vi "HeatFlow HW Conf Load.vi"(11 "Conf File":path) -> (0 "error out":errorcluster, 3 "HeatFlow HW Cfg":T1)   [LabVIEW 2019, in "Acquisition.lvlib"]
uses:
  Acquisition.lvlib
  HeatFlow HW Cfg.ctl
  HeatFlow Acq States.ctl
  <vilib>/Utility/config.llb/Read Key (Boolean).vi
  <vilib>/Utility/config.llb/Read Key (Double).vi
  <vilib>/Utility/config.llb/Read Key (String).vi
  <vilib>/Utility/config.llb/NI_LVConfig.lvlib
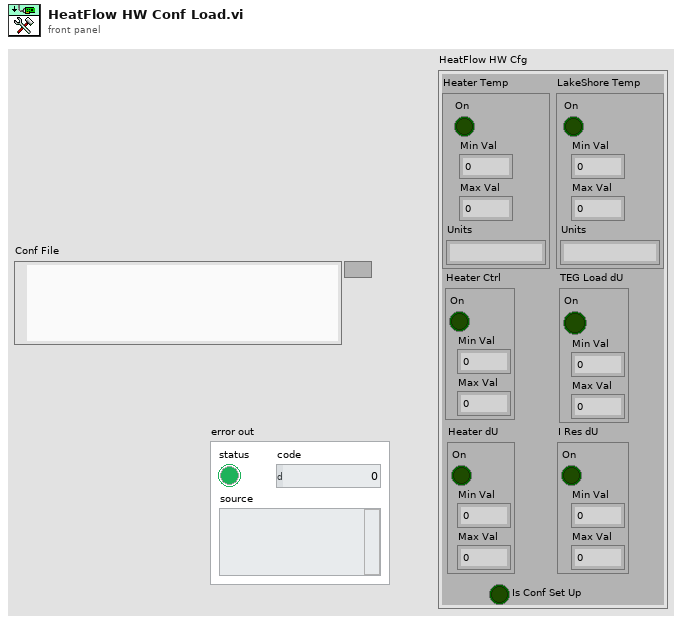
[diagram p1: front panel]
types:
  T1 = typedef "Acquisition.lvlib/HeatFlow HW Cfg.ctl" = cluster{"Heater Temp":cluster{"On":bool, "Min Val":dbl, "Max Val":dbl, "Units":string}, "LakeShore Temp":cluster{"On":bool, "Min Val":dbl, "Max Val":dbl, "Units":string}, "Heater Ctrl":cluster{"On":bool, "Min Val":dbl, "Max Val":dbl}, "TEG Load dU":cluster{"On":bool, "Min Val":dbl, "Max Val":dbl}, "Heater dU":cluster{"On":bool, "Min Val":dbl, "Max Val":dbl}, "I Res dU":cluster{"On":bool, "Min Val":dbl, "Max Val":dbl}, "Is Conf Set Up":bool}
  T2 = typedef "Acquisition.lvlib/HeatFlow Acq States.ctl" = enum16{"Start", "--- Control ---", "HeaterTemp", "DoControl?", "HeaterCtrl", "--- Readings ---", "DoReadings?", "I_Res_dU", "LakeShoreTemp", "Heater_dU", "TEG_Load_dU", "Calculations", "End"}
  T3 = typedef "NI_LVConfig.lvlib/Config Data RefNum.ctl" = refnum<k1>
  T4 = cluster{"On":bool, "Min Val":dbl, "Max Val":dbl, "Units":string}
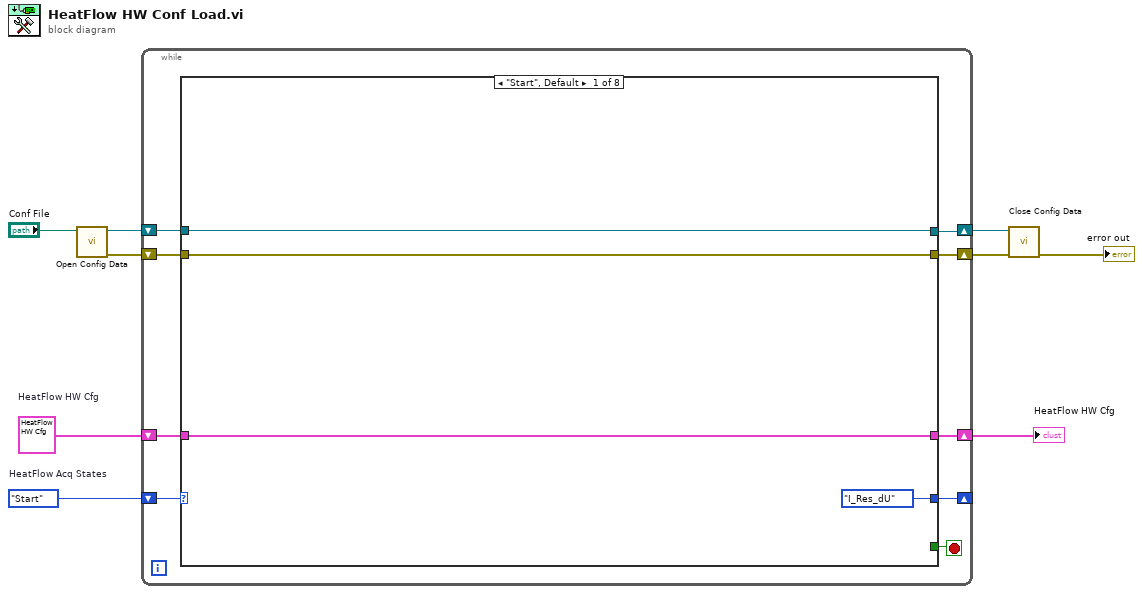
[diagram p0: block diagram]
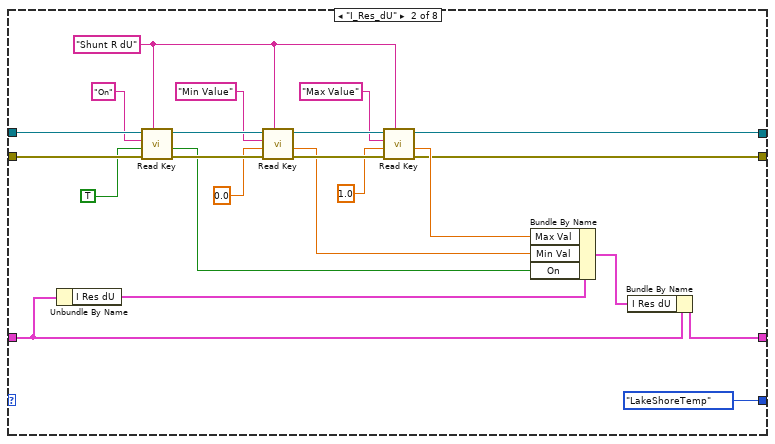
[diagram p2: hidden frame]
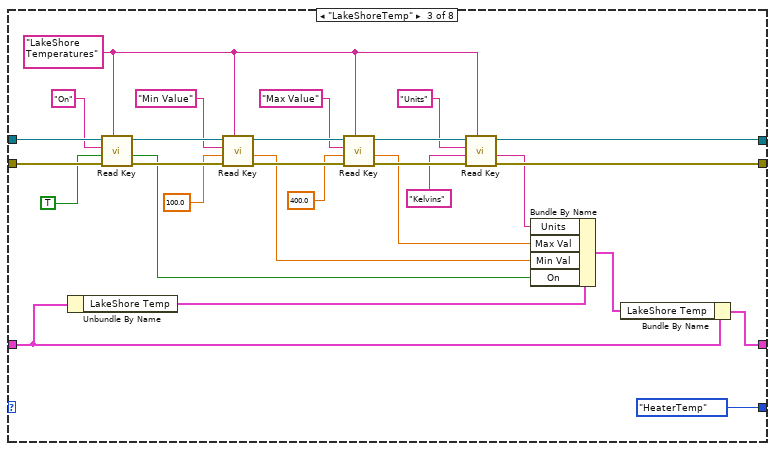
[diagram p3: hidden frame]
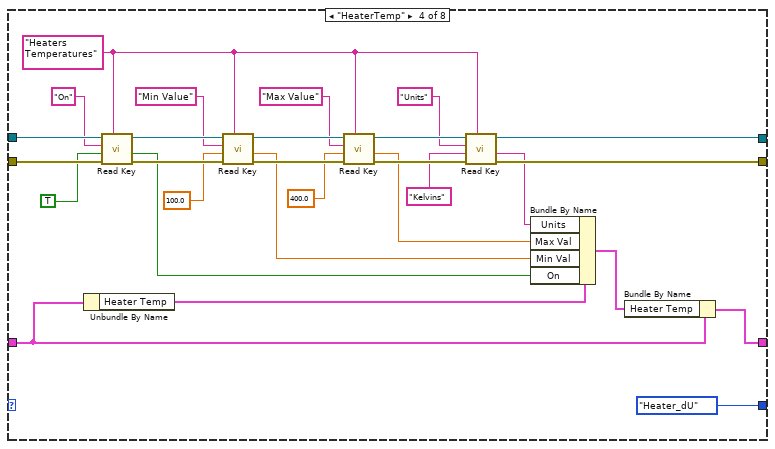
[diagram p4: hidden frame]
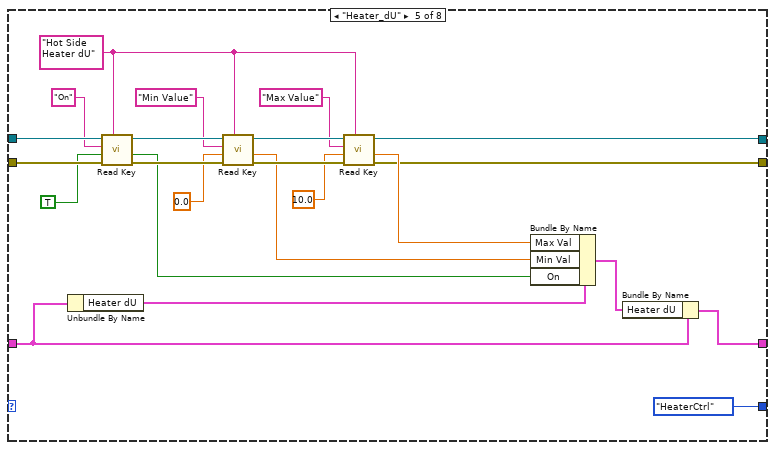
[diagram p5: hidden frame]
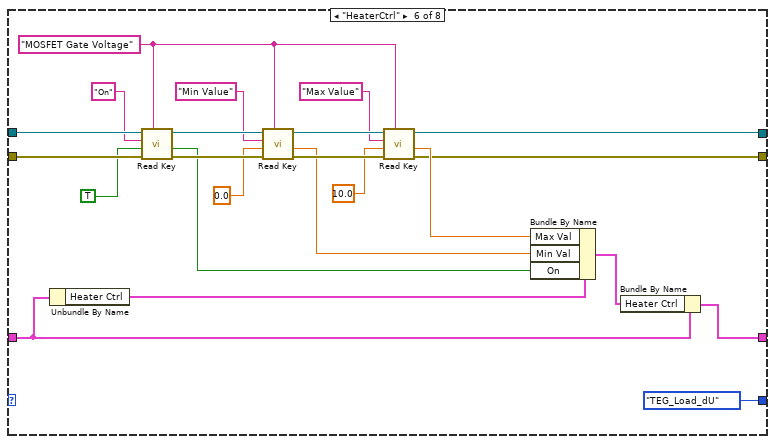
[diagram p6: hidden frame]
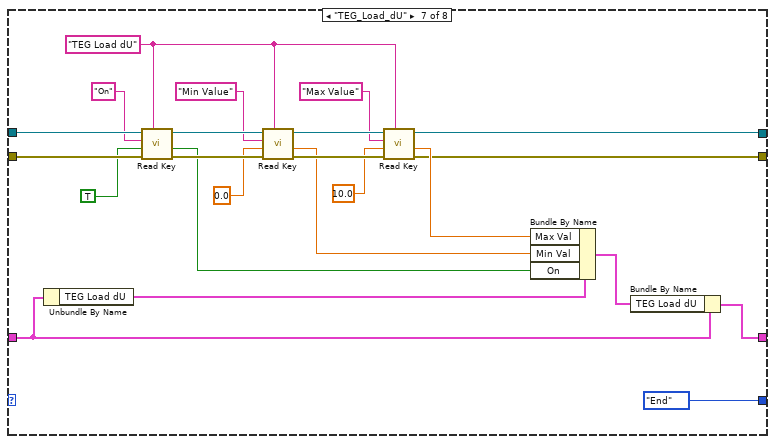
[diagram p7: hidden frame]
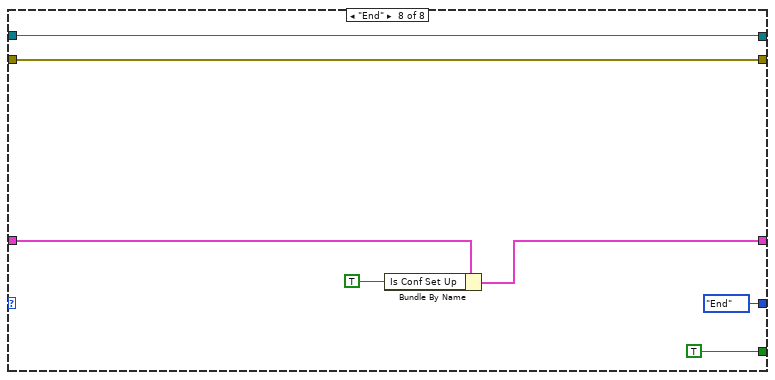
[diagram p8: hidden frame]
diagram:
  w5 = T1 {"Heater Temp"={"On"=FALSE, "Min Val"=0.0, "Max Val"=0.0, "Units"=""}, "LakeShore Temp"={"On"=FALSE, "Min Val"=0.0, "Max Val"=0.0, "Units"=""}, "Heater Ctrl"={"On"=FALSE, "Min Val"=0.0, "Max Val"=0.0}, "TEG Load dU"={"On"=FALSE, "Min Val"=0.0, "Max Val"=0.0}, "Heater dU"={"On"=FALSE, "Min Val"=0.0, "Max Val"=0.0}, "I Res dU"={"On"=FALSE, "Min Val"=0.0, "Max Val"=0.0}, "Is Conf Set Up"=FALSE}  # HeatFlow HW Cfg
  w9 = HeatFlow_Acq_States."Start"  # HeatFlow Acq States
  n1 = call <vilib>:"Open Config Data.vi"("configuration file path"="Conf File") -> ("error out"=w3:errorcluster, "refnum"=w2:T3)  [unwired: 8 in, 1 out]
  n2 = while {
    shift-right: [w17] -> _
    shift-left: w9 -> [w18]
    shift-right: [w11] -> w4
    shift-left: w5 -> [w15]
    shift-right: [w13] -> w8
    shift-left: w3 -> [w14]
    shift-right: [w12] -> w7
    shift-left: w2 -> [w16]
    stop <- w10 stop-if-true
    n3 = case shown="\"Start\", Default" w18 {
      tunnel: [HeatFlow_Acq_States."I_Res_dU" ("Measurement States") HeatFlow_Acq_States."LakeShoreTemp" ("Measurement States") HeatFlow_Acq_States."HeaterTemp" ("Measurement States") HeatFlow_Acq_States."Heater_dU" ("Measurement States") HeatFlow_Acq_States."HeaterCtrl" ("Measurement States") HeatFlow_Acq_States."TEG_Load_dU" ("Measurement States") HeatFlow_Acq_States."End" ("Measurement States") HeatFlow_Acq_States."End" ("Measurement States")] -> w17
      tunnel: w16 -> [w19 w44 w72 w100 w123 w146 w169 w173]
      tunnel: w15 -> [w21 w30 w52 w80 w109 w132 w155 w176]
      tunnel: w14 -> [w20 w43 w71 w99 w122 w145 w168 w172]
      tunnel: [w20 w23 w63 w91 w102 w125 w148 w172] -> w13
      tunnel: [w19 w24 w67 w95 w103 w126 w149 w173] -> w12
      tunnel: [w21 w28 w50 w78 w107 w130 w153 w175] -> w11
      tunnel: [_ _ _ _ _ _ _ TRUE] -> w10
      frame "Start", Default {
      }
      frame "I_Res_dU" {
        w38 = "Shunt R dU" ("section")
        n4 = Unbundle By Name(w30) -> ("I Res dU"=w34:cluster{"On":bool, "Min Val":dbl, "Max Val":dbl})
        n5 = call-poly <vilib>:"Read Key.vi"("section"=w38, "error in (no error)"=w43, "default value"=TRUE, "key"="On", "refnum"=w44) -> ("error out"=w40:errorcluster, "value"=w33:bool, "refnum out"=w42:T3)  [unwired: 3 in, 1 out]
        n6 = call-poly <vilib>:"Read Key.vi"("section"=w38, "error in (no error)"=w40, "default value"=0.0, "key"="Min Value", "refnum"=w42) -> ("error out"=w39:errorcluster, "value"=w32:dbl, "refnum out"=w41:T3)  [unwired: 3 in, 1 out]
        n7 = call-poly <vilib>:"Read Key.vi"("section"=w38, "error in (no error)"=w39, "default value"=1.0, "key"="Max Value", "refnum"=w41) -> ("error out"=w23:errorcluster, "value"=w31:dbl, "refnum out"=w24:T3)  [unwired: 3 in, 1 out]
        n8 = Bundle By Name(cluster=w34, "Max Val"=w31, "Min Val"=w32, "On"=w33) -> (w29:cluster{"On":bool, "Min Val":dbl, "Max Val":dbl})
        n9 = Bundle By Name(cluster=w30, "I Res dU"=w29) -> (w28:T1)
      }
      frame "LakeShoreTemp" {
        w62 = "LakeShore Temperatures" ("section")
        n10 = Unbundle By Name(w52) -> ("LakeShore Temp"=w57:T4)
        n11 = call-poly <vilib>:"Read Key.vi"("section"=w62, "error in (no error)"=w71, "default value"=TRUE, "key"="On", "refnum"=w72) -> ("error out"=w66:errorcluster, "value"=w56:bool, "refnum out"=w70:T3)  [unwired: 3 in, 1 out]
        n12 = call-poly <vilib>:"Read Key.vi"("section"=w62, "error in (no error)"=w66, "default value"=100.0, "key"="Min Value", "refnum"=w70) -> ("error out"=w65:errorcluster, "value"=w55:dbl, "refnum out"=w69:T3)  [unwired: 3 in, 1 out]
        n13 = call-poly <vilib>:"Read Key.vi"("section"=w62, "error in (no error)"=w65, "default value"=400.0, "key"="Max Value", "refnum"=w69) -> ("error out"=w64:errorcluster, "value"=w54:dbl, "refnum out"=w68:T3)  [unwired: 3 in, 1 out]
        n14 = call-poly <vilib>:"Read Key.vi"("section"=w62, "error in (no error)"=w64, "default value"="Kelvins", "key"="Units", "refnum"=w68) -> ("error out"=w63:errorcluster, "value"=w53:string, "refnum out"=w67:T3)  [unwired: 3 in, 1 out]
        n15 = Bundle By Name(cluster=w57, "Units"=w53, "Max Val"=w54, "Min Val"=w55, "On"=w56) -> (w51:T4)
        n16 = Bundle By Name(cluster=w52, "LakeShore Temp"=w51) -> (w50:T1)
      }
      frame "HeaterTemp" {
        w90 = "Heaters Temperatures" ("section")
        n17 = Unbundle By Name(w80) -> ("Heater Temp"=w85:T4)
        n18 = call-poly <vilib>:"Read Key.vi"("section"=w90, "error in (no error)"=w99, "default value"=TRUE, "key"="On", "refnum"=w100) -> ("error out"=w94:errorcluster, "value"=w84:bool, "refnum out"=w98:T3)  [unwired: 3 in, 1 out]
        n19 = call-poly <vilib>:"Read Key.vi"("section"=w90, "error in (no error)"=w94, "default value"=100.0, "key"="Min Value", "refnum"=w98) -> ("error out"=w93:errorcluster, "value"=w83:dbl, "refnum out"=w97:T3)  [unwired: 3 in, 1 out]
        n20 = call-poly <vilib>:"Read Key.vi"("section"=w90, "error in (no error)"=w93, "default value"=400.0, "key"="Max Value", "refnum"=w97) -> ("error out"=w92:errorcluster, "value"=w82:dbl, "refnum out"=w96:T3)  [unwired: 3 in, 1 out]
        n21 = call-poly <vilib>:"Read Key.vi"("section"=w90, "error in (no error)"=w92, "default value"="Kelvins", "key"="Units", "refnum"=w96) -> ("error out"=w91:errorcluster, "value"=w81:string, "refnum out"=w95:T3)  [unwired: 3 in, 1 out]
        n22 = Bundle By Name(cluster=w85, "Units"=w81, "Max Val"=w82, "Min Val"=w83, "On"=w84) -> (w79:T4)
        n23 = Bundle By Name(cluster=w80, "Heater Temp"=w79) -> (w78:T1)
      }
      frame "Heater_dU" {
        w117 = "Hot Side Heater dU" ("section")
        n24 = Unbundle By Name(w109) -> ("Heater dU"=w113:cluster{"On":bool, "Min Val":dbl, "Max Val":dbl})
        n25 = call-poly <vilib>:"Read Key.vi"("section"=w117, "error in (no error)"=w122, "default value"=TRUE, "key"="On", "refnum"=w123) -> ("error out"=w119:errorcluster, "value"=w112:bool, "refnum out"=w121:T3)  [unwired: 3 in, 1 out]
        n26 = call-poly <vilib>:"Read Key.vi"("section"=w117, "error in (no error)"=w119, "default value"=0.0, "key"="Min Value", "refnum"=w121) -> ("error out"=w118:errorcluster, "value"=w111:dbl, "refnum out"=w120:T3)  [unwired: 3 in, 1 out]
        n27 = call-poly <vilib>:"Read Key.vi"("section"=w117, "error in (no error)"=w118, "default value"=10.0, "key"="Max Value", "refnum"=w120) -> ("error out"=w102:errorcluster, "value"=w110:dbl, "refnum out"=w103:T3)  [unwired: 3 in, 1 out]
        n28 = Bundle By Name(cluster=w113, "Max Val"=w110, "Min Val"=w111, "On"=w112) -> (w108:cluster{"On":bool, "Min Val":dbl, "Max Val":dbl})
        n29 = Bundle By Name(cluster=w109, "Heater dU"=w108) -> (w107:T1)
      }
      frame "HeaterCtrl" {
        w140 = "MOSFET Gate Voltage" ("section")
        n30 = Unbundle By Name(w132) -> ("Heater Ctrl"=w136:cluster{"On":bool, "Min Val":dbl, "Max Val":dbl})
        n31 = call-poly <vilib>:"Read Key.vi"("section"=w140, "error in (no error)"=w145, "default value"=TRUE, "key"="On", "refnum"=w146) -> ("error out"=w142:errorcluster, "value"=w135:bool, "refnum out"=w144:T3)  [unwired: 3 in, 1 out]
        n32 = call-poly <vilib>:"Read Key.vi"("section"=w140, "error in (no error)"=w142, "default value"=0.0, "key"="Min Value", "refnum"=w144) -> ("error out"=w141:errorcluster, "value"=w134:dbl, "refnum out"=w143:T3)  [unwired: 3 in, 1 out]
        n33 = call-poly <vilib>:"Read Key.vi"("section"=w140, "error in (no error)"=w141, "default value"=10.0, "key"="Max Value", "refnum"=w143) -> ("error out"=w125:errorcluster, "value"=w133:dbl, "refnum out"=w126:T3)  [unwired: 3 in, 1 out]
        n34 = Bundle By Name(cluster=w136, "Max Val"=w133, "Min Val"=w134, "On"=w135) -> (w131:cluster{"On":bool, "Min Val":dbl, "Max Val":dbl})
        n35 = Bundle By Name(cluster=w132, "Heater Ctrl"=w131) -> (w130:T1)
      }
      frame "TEG_Load_dU" {
        w163 = "TEG Load dU" ("section")
        n36 = Unbundle By Name(w155) -> ("TEG Load dU"=w159:cluster{"On":bool, "Min Val":dbl, "Max Val":dbl})
        n37 = call-poly <vilib>:"Read Key.vi"("section"=w163, "error in (no error)"=w168, "default value"=TRUE, "key"="On", "refnum"=w169) -> ("error out"=w165:errorcluster, "value"=w158:bool, "refnum out"=w167:T3)  [unwired: 3 in, 1 out]
        n38 = call-poly <vilib>:"Read Key.vi"("section"=w163, "error in (no error)"=w165, "default value"=0.0, "key"="Min Value", "refnum"=w167) -> ("error out"=w164:errorcluster, "value"=w157:dbl, "refnum out"=w166:T3)  [unwired: 3 in, 1 out]
        n39 = call-poly <vilib>:"Read Key.vi"("section"=w163, "error in (no error)"=w164, "default value"=10.0, "key"="Max Value", "refnum"=w166) -> ("error out"=w148:errorcluster, "value"=w156:dbl, "refnum out"=w149:T3)  [unwired: 3 in, 1 out]
        n40 = Bundle By Name(cluster=w159, "Max Val"=w156, "Min Val"=w157, "On"=w158) -> (w154:cluster{"On":bool, "Min Val":dbl, "Max Val":dbl})
        n41 = Bundle By Name(cluster=w155, "TEG Load dU"=w154) -> (w153:T1)
      }
      frame "End" {
        n42 = Bundle By Name(cluster=w176, "Is Conf Set Up"=TRUE) -> (w175:T1)
      }
    }
  }
  "HeatFlow HW Cfg" <- w4
  n43 = call <vilib>:"Close Config Data.vi"("error in (no error)"=w8, "refnum"=w7) -> ("error out"=→"error out":errorcluster)  [unwired: 8 in, 1 out]
